vi "Update Instrument Calibration.vi"(8 "error in (no error)":errorcluster, 11 "PicoScope 3000a in":refnum<class "PicoScope 3000a.lvclass">) -> (0 "error out":errorcluster, 3 "PicoScope 3000a out":refnum<class "PicoScope 3000a.lvclass">)   [LabVIEW 2018, in "PicoScope 3000a.lvlib" / "PicoScope 3000a.lvclass"]
uses:
  PicoScope 3000a.lvclass
  PicoScope 3000a.lvclass/PicoScope 3000a.ctl
  PPLs/Oscilloscope/Parent/Oscilloscope.lvlibp/Oscilloscope.lvclass
  PPLs/Oscilloscope/Parent/Configuration.lvlibp/Configuration.lvclass
  C:/Projects/LabVIEW/PPLs/Oscilloscope/Parent/Oscilloscope.lvlibp/Oscilloscope.lvclass
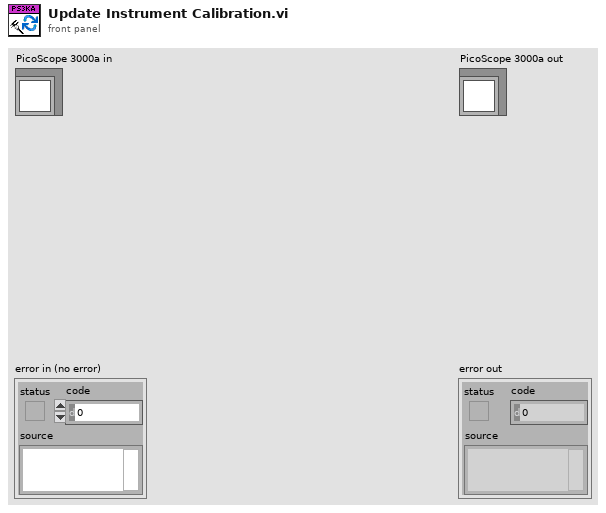
[diagram p1: front panel]
types:
  T1 = cluster{"Driver Version":string, "USB Version":string, "Hardware":string, "Variant":string, "Batch and Serial":string, "Cal Date":string, "Kernel Version":string, "Digital HW Version":string, "Analogue HW Version":string, "MSO":bool, "Number of channels":i16}
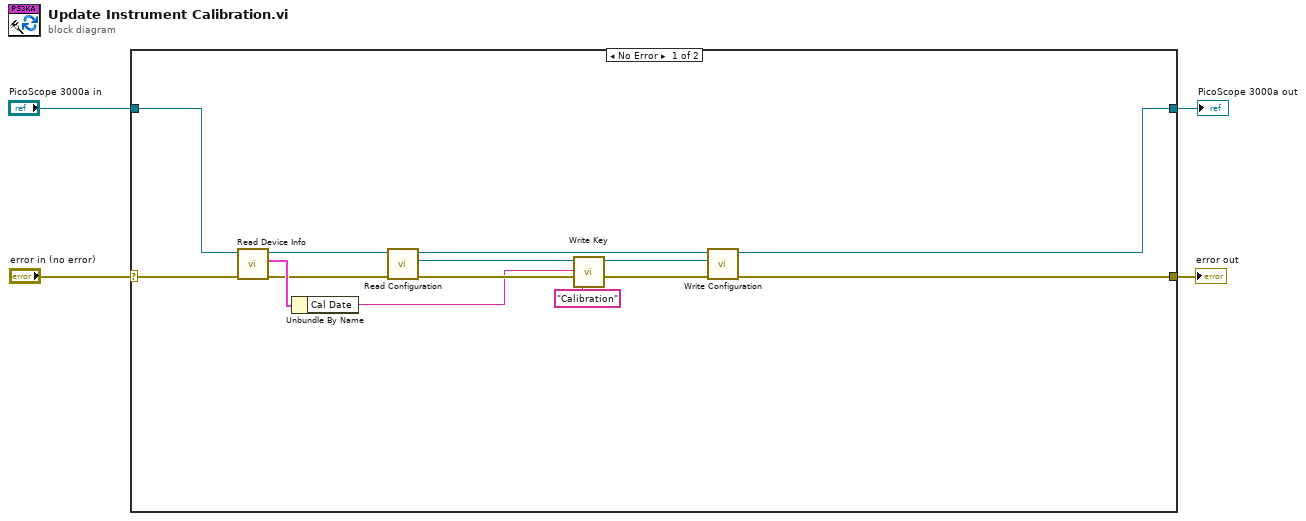
[diagram p0: block diagram]
diagram:
  n1 = case shown="No Error" "error in (no error)" {
    selector: "error in (no error)" -> [w18 w20]
    tunnel: [w5 w20] -> w3
    tunnel: [w6 w19] -> w1
    tunnel: "PicoScope 3000a in" -> [w17 w19]
    frame No Error {
      n2 = call "Read Device Info.vi"("error in (no error)"=w18, "PicoScope 3000a in"=w17) -> ("error out"=w13:errorcluster, "Device Info"=w16:T1, "PicoScope 3000a out"=w15:refnum<class "PicoScope 3000a.lvclass">)  [unwired: 7 in]
      n3 = Unbundle By Name(w16) -> ("Cal Date"=w10:string)
      n4 = call "Read Configuration.vi"("error in (no error)"=w13, "Oscilloscope in"=w15) -> ("error out"=w12:errorcluster, "Configuration"=w14:refnum<class "Configuration.lvclass">, "Oscilloscope out"=w8:refnum<class "PicoScope 3000a.lvclass">)  [unwired: 7 in]
      n5 = call "Write Key.vi"("error in"=w12, "value"=w10, "key"="Calibration", "Configuration in"=w14) -> ("error out"=w7:errorcluster, "Configuration out"=w9:refnum<class "Configuration.lvclass">)  [unwired: 6 in]
      n6 = call "Write Configuration.vi"("error in (no error)"=w7, "Configuration"=w9, "Oscilloscope in"=w8) -> ("error out"=w5:errorcluster, "Oscilloscope out"=w6:refnum<class "PicoScope 3000a.lvclass">)  [unwired: 7 in]
    }
    frame Error {
    }
  }
  "error out" <- w3
  "PicoScope 3000a out" <- w1
